vi "1A.1 WriteToFIFOPort1.vi"() -> ()   [LabVIEW 2011]
doc: "Elizabeth Mahon\nSets properties of sensor in port 1 of serial port (in this case, the compass), reads value from sensor, and puts it into a FIFO to be read on the cRIO.\nAlso lets us blink the light on the cRIO as a test.\nALWAYS run it from the FPGA target, not the folder - it doesn't work if you try to run it from the folder.\nIt works!\n\nDeprecated now due to the new sensor. I'm keeping it here so we can reference it if it turns out we need to read from the FPGA."
uses:
  <vilib>/rvi/DataTransferAndStorage/Container/XNode/niFpgaContainer.xnode
  <vilib>/eio/EIOMethodNode/EIOMethodNode.xnode
  <vilib>/rvi/eio/common/nirviEmuTemplateMethod_errors.vi
  <vilib>/eio/EIONode/EIONode.xnode
  <vilib>/eio/EIOPropertyNode/EIOPropertyNode.xnode
  <vilib>/LabVIEW Targets/FPGA/cRIO/shared/nicrio_ModuleControls/nicrio_cRIO-9871_BaudRateEnum.ctl
  <vilib>/LabVIEW Targets/FPGA/cRIO/shared/nicrio_ModuleControls/nicrio_cRIO-9871_DataBitsEnum.ctl
  <vilib>/rvi/interface/RandomDataEmulation/nirviRandomDataFpgaReadWriteTemplate.vi
  <vilib>/rvi/eio/common/nirviEmuTemplatePropertyGet_errors.vi
  <vilib>/rvi/eio/common/nirviEmuTemplatePropertyGet_noerrors.vi
  <vilib>/rvi/eio/common/nirviEmuTemplatePropertySet_errors.vi
  <vilib>/rvi/eio/common/nirviEmuTemplatePropertySet_noerrors.vi
panel:
  in  "We probably want it to be able to be stopped from the global, too.":bool
  in  "FPGA LED":bool
  in  "stoplight":bool
  out "Numeric":i32
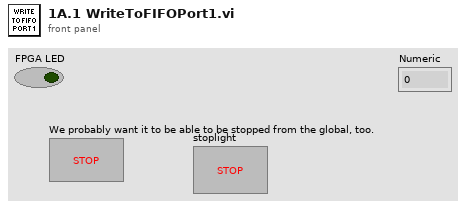
[diagram p1: front panel]
types:
  T1 = typedef "nicrio_cRIO-9871_DataBitsEnum.ctl" = enum8{"5", "6", "7", "8"}
  T2 = typedef "nicrio_cRIO-9871_BaudRateEnum.ctl" = enum16{"75 bps", "110 bps", "134 bps", "150 bps", "300 bps", "600 bps", "1200 bps", "1800 bps", "2400 bps", "4800 bps", "7200 bps", "9600 bps", "14.4 kbps", "19.2 kbps", "28.8 kbps", "38.4 kbps", "57.6 kbps", "115.2 kbps", "230.4 kbps", "460.8 kbps", "921.6 kbps"}
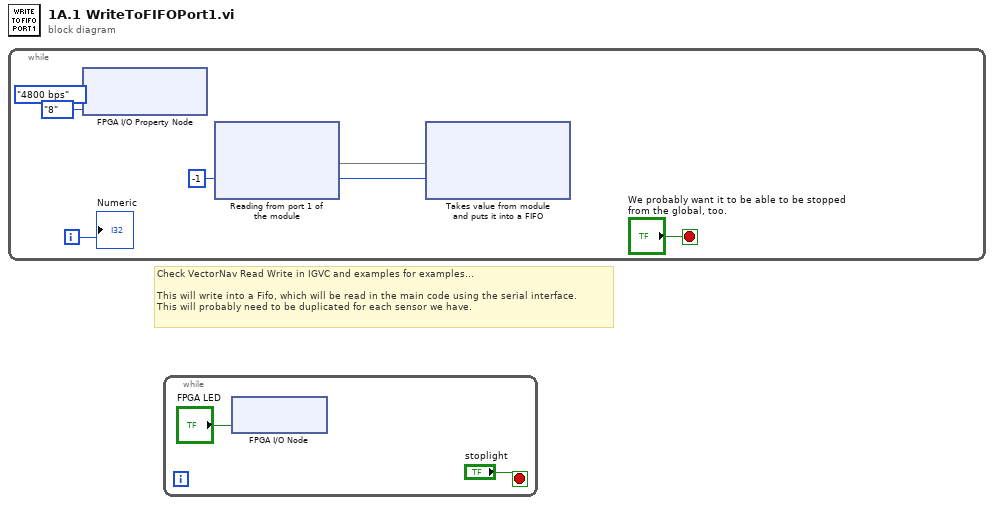
[diagram p0: block diagram]
diagram:
  # "Check VectorNav Read Write in IGVC and examples for examples...\n\nThis will write into a Fifo, which will be read in the main code using the serial interface.\nThis will probably need to be duplicated for each sensor we have."
  n1 = while {
    i -> [w5]
    stop <- "We probably want it to be able to be stopped from the global, too." stop-if-true
    w1 = -1 ("Timeout (ms)")
    n2 = xnode "FPGA I/O Property Node"("Baud Rate"=nicrio_cRIO-9871_BaudRateEnum."4800 bps", "Data Bits"=nicrio_cRIO-9871_DataBitsEnum."8") -> ()  [unwired: 1 in, 1 out]
    n3 = xnode "Reading from port 1 of the module"("Timeout (ms)"=w1) -> ("Data"=w6)  [unwired: 1 in, 2 out]
    n4 = xnode "Takes value from module and puts it into a FIFO"("Element"=w6, "Timeout"=w1) -> ()  [unwired: 1 in, 2 out]
    "Numeric" <- w5
  }
  n5 = while {
    stop <- "stoplight" stop-if-true
    n6 = xnode "FPGA I/O Node"("FPGA LED"="FPGA LED") -> ()  [unwired: 1 in, 1 out]
  }
